vi "Read.vi"(8 "error in (no error)":errorcluster, 9 "Timeout":u32, 10 "Last message":refnum<class "BaseMessage.lvclass">, 11 "BaseReader in":refnum<class "BaseReader.lvclass">) -> (0 "error out":errorcluster, 1 "isAck?":bool, 2 "Responses":T1[](array[typedef]), 3 "BaseReader out":refnum<class "BaseReader.lvclass">)   [LabVIEW 2013, in "BaseReader.lvclass"]
doc: "Read a message from the remote destination"
uses:
  BaseReader.lvclass
  Message/BaseMessage/BaseMessage.lvclass
  response.ctl
  driver_status.ctl
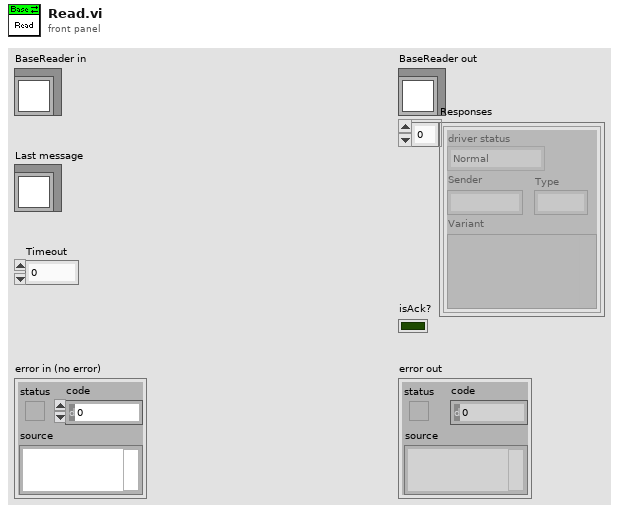
[diagram p1: front panel]
types:
  T1 = typedef "response.ctl" = cluster{"driver status":T2, "Sender":string, "Type":i32, "Variant":variant}
  T2 = typedef "driver_status.ctl" = enum16{"Normal", "Startup", "Connection lost", "Reconnected", "Timeout", "Idle", "Busy"}
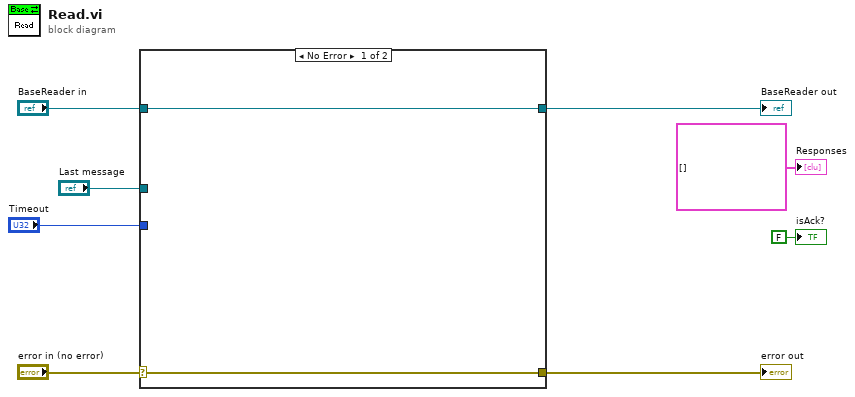
[diagram p0: block diagram]
diagram:
  n1 = case shown="No Error" "error in (no error)" {
    selector: "error in (no error)" -> [w9 w12]
    tunnel: [w9 w12] -> w7
    tunnel: [w10 w11] -> w5
    tunnel: "BaseReader in" -> [w10 w11]
    tunnel: "Last message" -> [_ _]
    tunnel: "Timeout" -> [_ _]
    frame No Error {
    }
    frame Error {
    }
  }
  "error out" <- w7
  "BaseReader out" <- w5
  "Responses" <- T1[] [] ("Responses")
  "isAck?" <- FALSE ("isAck?")
